vi "CalibrationState.vi"() -> ()   [LabVIEW 2013]
panel:
  in  "CalibrationState":cluster{bool, "CalibrationState":u32}
  # "CalibrationDone"
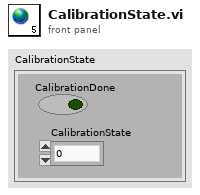
[diagram p1: front panel]
diagram:
